vi "Measurement UI.vi"() -> ()   [LabVIEW 2021, in "adc_chToChIsolationMeasurement.lvlib"]
uses:
  adc_chToChIsolationMeasurement.lvlib
panel:
  in  "MeasGraphs":T1(tab)
  out "FreqDomainGraph":cluster{"f0":dbl, "df":dbl, "Spectrum":dbl[]}[](graph) caption="AC"
  out "TimeDomainGraph":waveform(dbl)[](graph) caption="AC"
  out "CrosstalkGraph":T2(graph)
  out "Time domain plot size":i32
  out "Spectrum plot size":i32
  out "dt":dbl
  out "t0":dbl
  out "df":dbl
  out "f0":dbl
  out "Time domain":dbl[](array[numeric])
  out "Spectrum":dbl[](array[numeric])
  in  "Interferer channel resource name":string
  out "Frequency":dbl
  out "Crosstalk":dbl
  out "Victim channel name":string
  out "Crosstalk waveform":dbl[](array[numeric])
  out "Frequency waveform":dbl[](array[numeric])
  in  "Victim channel resource name":string
  in  "Digital capture resource name":string
  out "MeasTable":string[][](table)
  in  "Interferer channel channel":i32 caption="CHANNEL"
  in  "MeasSettingsOptions":i32(listbox)
  in  "Digital capture":string="Digital capture"
  in  "Analog source interferer":string="Analog source interferer"
  in  "Analog source victim":string="Analog source victim"
  in  "ADC parameters":string="ADC parameters"
  in  "MeasSettings":bool
  in  "Interferer sweep type":u32(ring) caption="SWEEP TYPE" items=["Linear", "Logarithmic"]
  in  "Interferer number of steps":i32=10 caption="NUMBER OF STEPS"
  in  "Interferer stop frequency":dbl=160000.0 caption="STOP FREQUENCY" format="%#_6pHz"
  in  "Interferer amplitude":dbl=-1.0 caption="AMPLITUDE" format="%#_6pdB"
  in  "Interferer start frequency":dbl=2000.0 caption="START FREQUENCY" format="%#_6pHz"
  in  "InterfererResourceName":refnum<k15> caption="RESOURCE NAME"
  in  "Interferer channels":i32[](array[numeric])=[2] caption="INTERFERER CHANNELS"
  in  "Digital capture samples":u32=80000 caption="NUMBER OF SAMPLES"
  in  "Victim channel":i32 caption="VICTIM CHANNEL" min=0 max=100 step=1
  in  "Full scale range":dbl=10.0 caption="FULL SCALE RANGE" format="%#_6pV"
  in  "Digital capture sample rate":dbl=800000.0 caption="SAMPLE RATE" format="%#_6pS/s"
  in  "Victim amplitude":dbl=-1.0 caption="AMPLITUDE" format="%#_6pdB"
  in  "Victim frequency":dbl=1000.0 caption="FREQUENCY" format="%#_6pHz"
  in  "VictimResourceName":tag caption="RESOURCE NAME"
  in  "DPIResourceName":refnum<k15> caption="RESOURCE NAME"
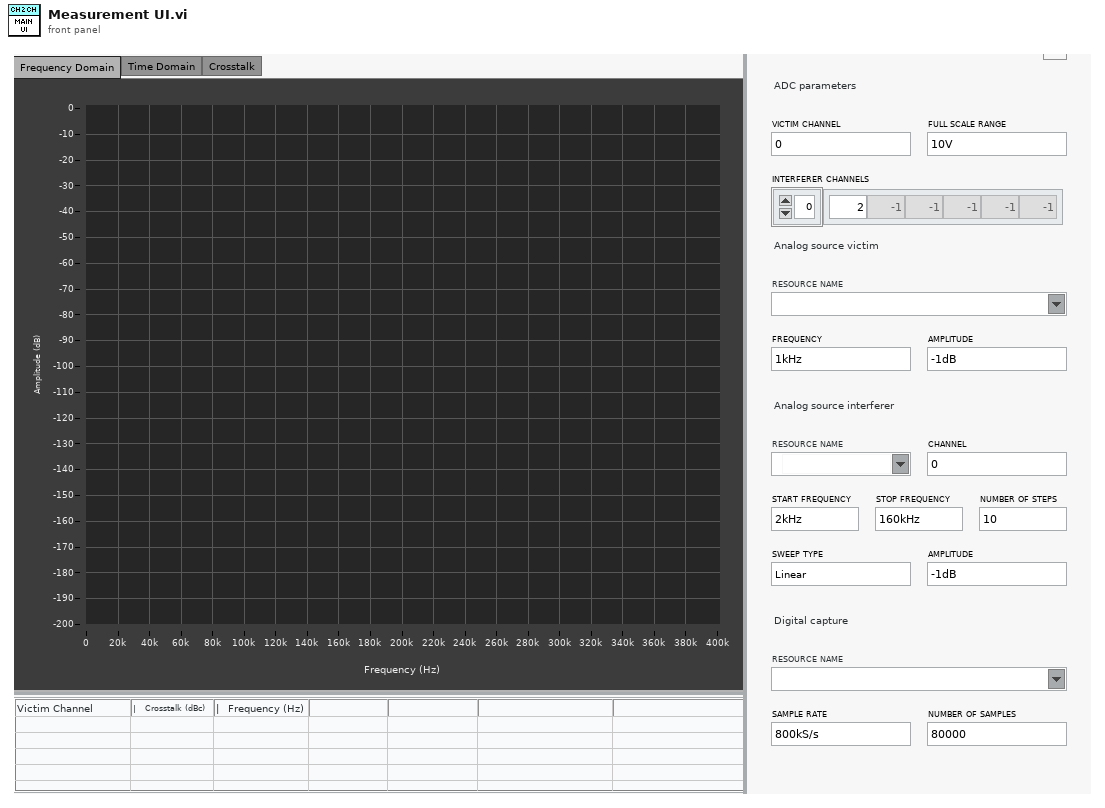
[diagram p1: front panel]
types:
  T1 = enum32{"Frequency Domain", "Time Domain", "Crosstalk", "Hidden Controls"}
  T2 = cluster{"Frequency waveform":dbl[], "Crosstalk waveform":dbl[]}
  T3 = enum16{"open", "replace", "create", "open or create", "replace or create", "replace or create with confirmation"}
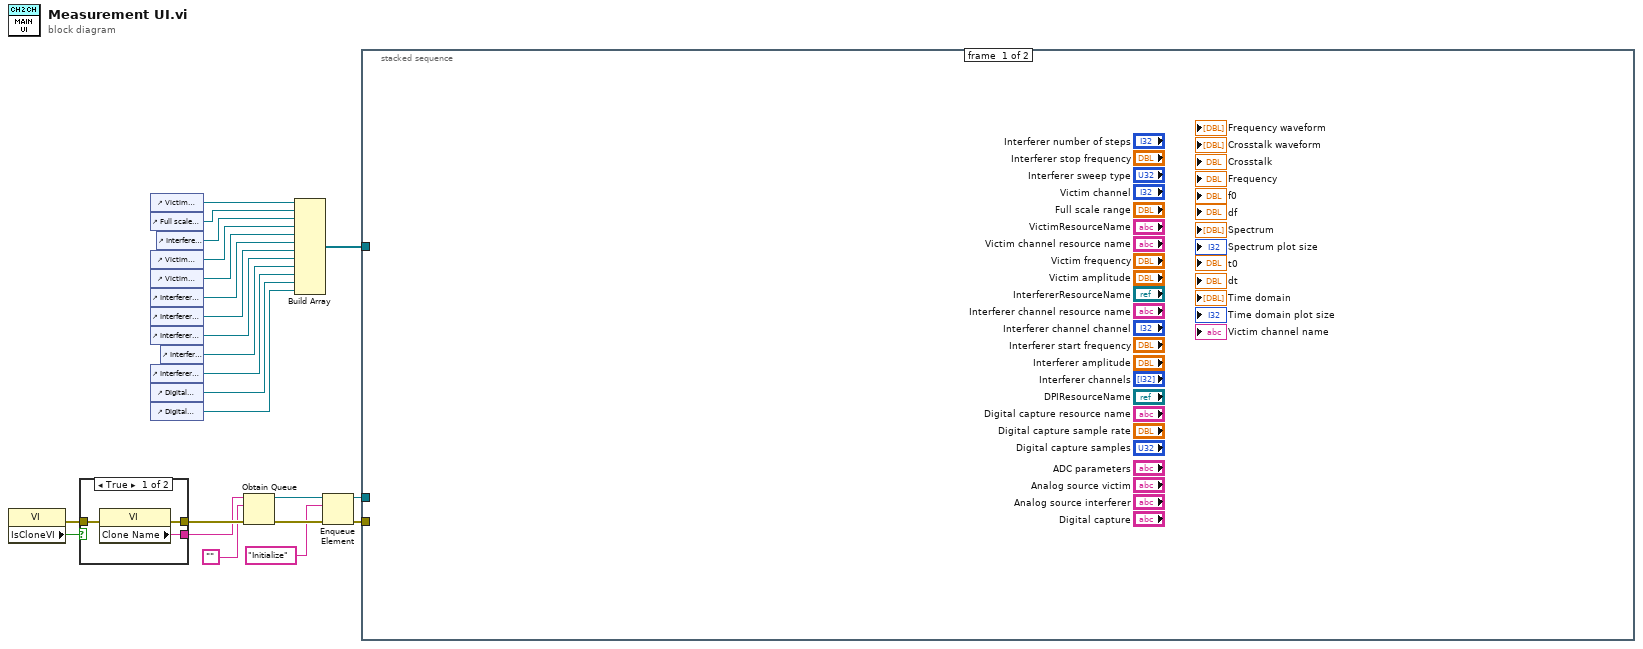
[diagram p0: block diagram]
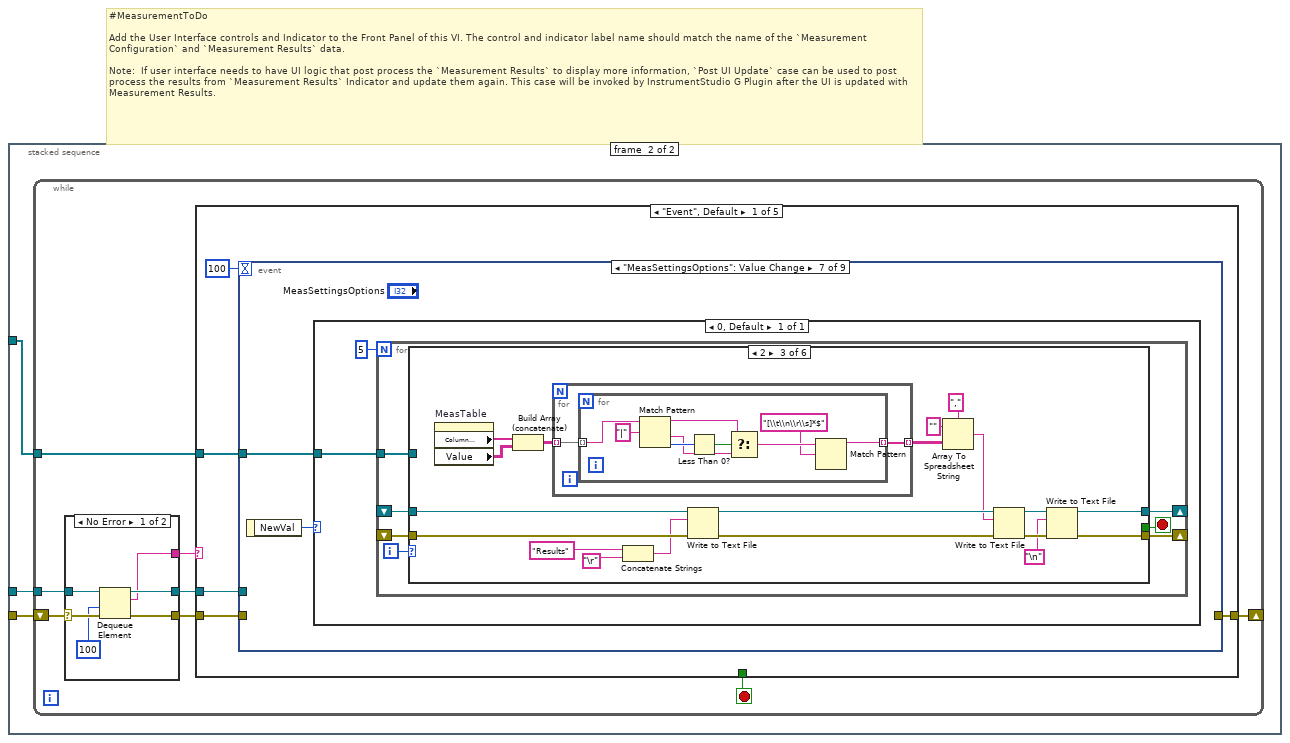
[diagram p2: hidden frame]
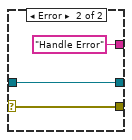
[diagram p3: hidden frame]
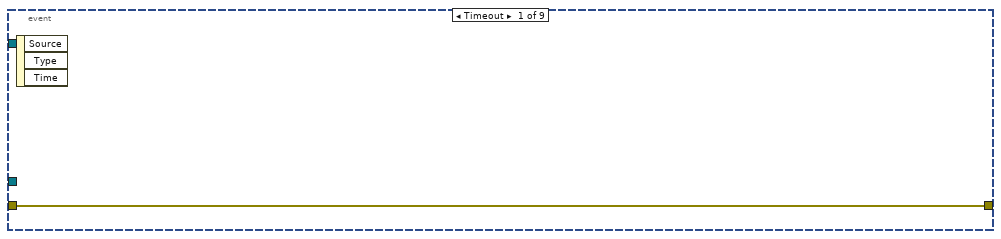
[diagram p4: hidden frame]
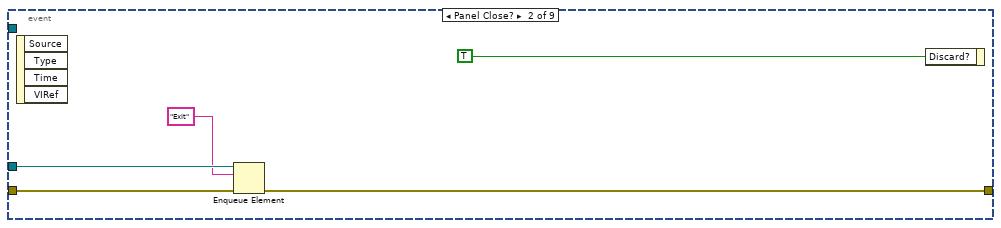
[diagram p5: hidden frame]
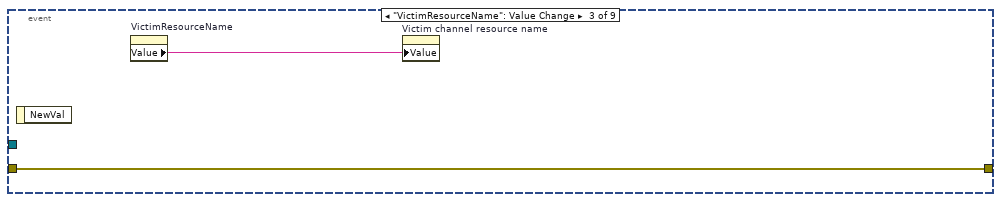
[diagram p6: hidden frame]
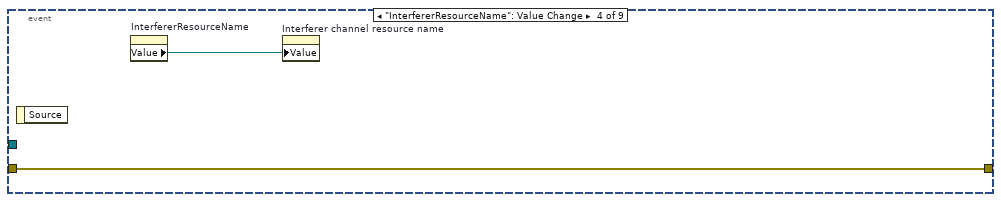
[diagram p7: hidden frame]
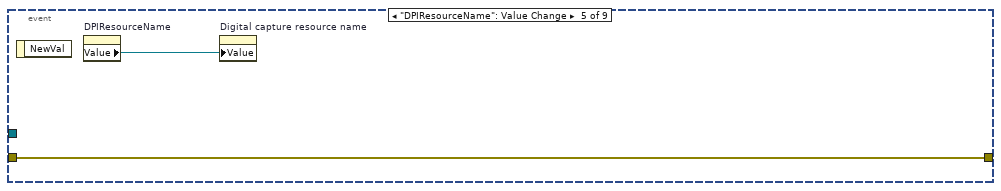
[diagram p8: hidden frame]
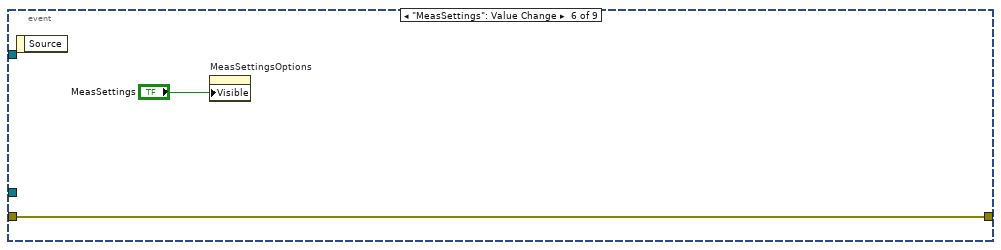
[diagram p9: hidden frame]
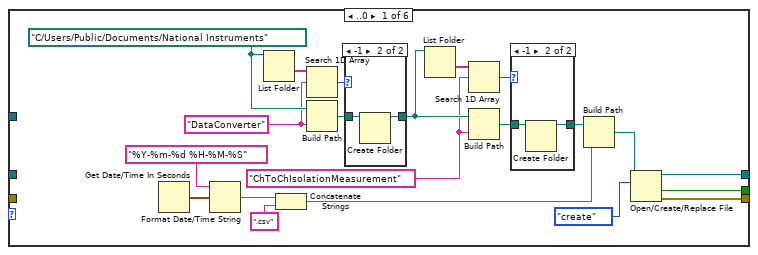
[diagram p10: hidden frame]
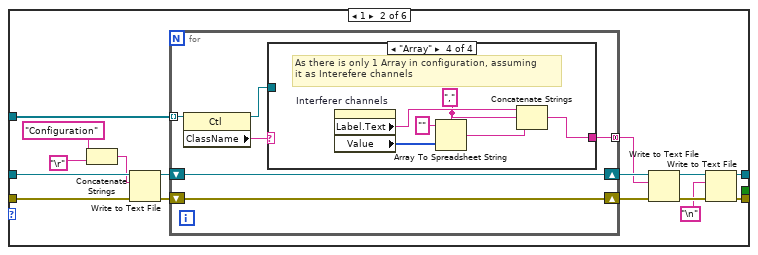
[diagram p13: hidden frame]
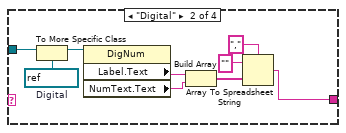
[diagram p15: hidden frame]
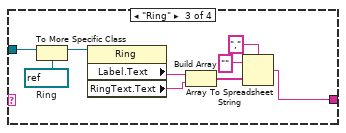
[diagram p16: hidden frame]
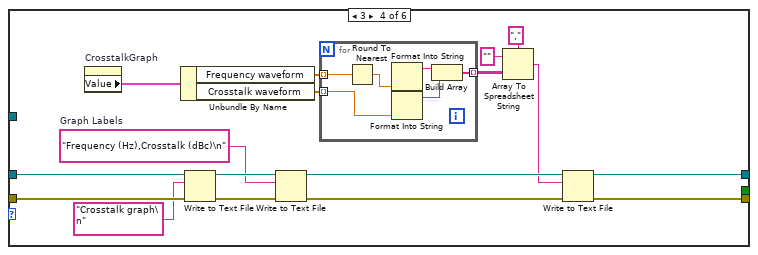
[diagram p17: hidden frame]
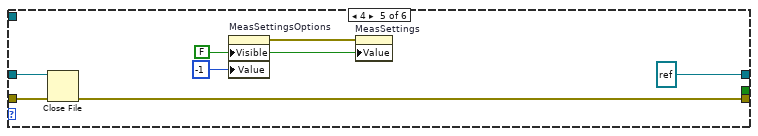
[diagram p18: hidden frame]
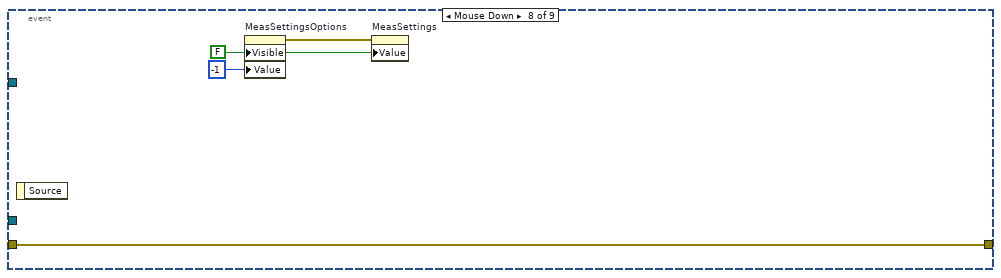
[diagram p20: hidden frame]
diagram:
  n1 = property class="VI"() -> (error out=w14:errorcluster, "IsCloneVI"=w15:bool)  [unwired: 2 in, 1 out]
  n2 = case shown="True" w15 {
    tunnel: [w26 w29] -> w23
    tunnel: [w25 w28] -> w22
    tunnel: w14 -> [w24 w27]
    frame True {
      n3 = property class="VI"(error in=w24) -> (error out=w26:errorcluster, "Clone Name"=w25:string)  [unwired: 1 in, 1 out]
    }
    frame False {
      n4 = property class="VI"(error in=w27) -> (error out=w29:errorcluster, "Name"=w28:string)  [unwired: 1 in, 1 out]
    }
  }
  n5 = control-ref of="Victim channel"() -> (w2:refnum<vi>)
  n6 = control-ref of="Full scale range"() -> (w3:refnum<vi>)
  n7 = control-ref of="Victim frequency"() -> (w5:refnum<vi>)
  n8 = control-ref of="Victim amplitude"() -> (w6:refnum<vi>)
  n9 = control-ref of="Interferer start frequency"() -> (w7:refnum<vi>)
  n10 = control-ref of="Interferer stop frequency"() -> (w8:refnum<vi>)
  n11 = control-ref of="Interferer number of steps"() -> (w9:refnum<vi>)
  n12 = control-ref of="Interferer amplitude"() -> (w11:refnum<vi>)
  n13 = control-ref of="Digital capture sample rate"() -> (w12:refnum<vi>)
  n14 = control-ref of="Digital capture samples"() -> (w13:refnum<vi>)
  n15 = control-ref of="Interferer channels"() -> (w4:refnum<vi>)
  n16 = control-ref of="Interferer sweep type"() -> (w10:refnum<vi>)
  n17 = Obtain Queue(name (unnamed)=w22, element data type="", error in (no error)=w23) -> (queue out=w19:refnum<queue>, error out=w21:errorcluster)  [unwired: 2 in, 1 out]
  n18 = Build Array(w2, w3, w4, w5, w6, w7, w8, w9, w10, w11, w12, w13) -> (w1:refnum<vi>[])
  n19 = Enqueue Element(queue=w19, element="Initialize", error in (no error)=w21) -> (queue out=w18:refnum<queue>, error out=w20:errorcluster)  [unwired: 1 in, 1 out]
  n20 = stacked-sequence {
    tunnel: w20 -> [_ w32]
    tunnel: w18 -> [_ w31]
    tunnel: w1 -> [_ w30]
    frame #0 {
    }
    frame #1 {
      # "#MeasurementToDo  \n\nAdd the User Interface controls and Indicator to the Front Panel of this VI. The control and indicator label name should match the name of the `Measurement Configuration` and `Measurement Results` data.\n\nNote:  If user interface needs to have UI logic that post process the `Measurement Results` to display more information, `Post UI Update` case can be used to post process the results from `Measurement Results` Indicator and update them again. This case will be invoked by InstrumentStudio G Plugin after the UI is updated with Measurement Results."
      n21 = while {
        shift-right: [w35] -> _
        shift-left: w32 -> [w40]
        tunnel: w31 -> [w38]
        tunnel: w30 -> [w33]
        stop <- w34 stop-if-true
        n22 = case shown="No Error" w40 {
          selector: w40 -> [w46 w49]
          tunnel: [w45 w49] -> w39
          tunnel: w38 -> [w44 w48]
          tunnel: [w43 w48] -> w37
          tunnel: [w42 "Handle Error"] -> w36
          frame No Error {
            n23 = Dequeue Element(queue=w44, timeout in ms (-1)=100, error in (no error)=w46) -> (queue out=w43:refnum<queue>, element=w42:string, error out=w45:errorcluster)  [unwired: 1 out]
          }
          frame Error {
          }
        }
        n24 = case shown="\"Event\", Default" w36 {
          tunnel: w39 -> [w53 w240 w268 w292 w293]
          tunnel: w37 -> [w51 _ _ w290 _]
          tunnel: [w54 w240 w268 w287 w293] -> w35
          tunnel: [_ _ _ TRUE _] -> w34
          tunnel: w33 -> [w50 _ _ _ _]
          frame "Event", Default {
            n25 = event shown="[6] \"MeasSettingsOptions\": Value Change" {
              selector: _ -> [_ _ _ _ _ _ _ _ _]
              dyn-events: _ -> [_ _ _ _ _ _ _ _ _]
              timeout: 100 -> [_ _ _ _ _ _ _ _ _]
              tunnel: [w55 w58 w62 w64 w65 w67 _ w218 w219] -> w54
              tunnel: w53 -> [w55 w59 w62 w64 w65 w67 _ w218 w219]
              tunnel: w51 -> [_ w57 _ _ _ _ _ _ _]
              tunnel: w50 -> [_ _ _ _ _ _ w69 _ _]
              event Timeout {
                n26 = event-data() -> ()  [unwired: 1 in, 3 out]
              }
              event Panel Close? {
                n27 = event-data() -> ()  [unwired: 1 in, 4 out]
                n28 = Enqueue Element(queue=w57, element="Exit", error in (no error)=w59) -> (error out=w58:errorcluster)  [unwired: 1 in, 2 out]
                n29 = event-data("Discard?"=TRUE) -> ()  [unwired: 1 in, 1 out]
              }
              event "VictimResourceName": Value Change {
                n30 = event-data() -> ()  [unwired: 1 in, 1 out]
                n31 = property on="VictimResourceName" class="DAQmxName"() -> ("Value"=w61:string)  [unwired: 2 in, 2 out]
                n32 = property on="Victim channel resource name" class="Str"("Value"=w61) -> ()  [unwired: 2 in, 2 out]
              }
              event "InterfererResourceName": Value Change {
                n33 = event-data() -> ()  [unwired: 1 in, 1 out]
                n34 = property on="InterfererResourceName" class="IVIName"() -> ("Value"=w63:refnum<k15>)  [unwired: 2 in, 2 out]
                n35 = property on="Interferer channel resource name" class="Str"("Value"=w63) -> ()  [unwired: 2 in, 2 out]
              }
              event "DPIResourceName": Value Change {
                n36 = event-data() -> ()  [unwired: 1 in, 1 out]
                n37 = property on="DPIResourceName" class="IVIName"() -> ("Value"=w66:refnum<k15>)  [unwired: 2 in, 2 out]
                n38 = property on="Digital capture resource name" class="Str"("Value"=w66) -> ()  [unwired: 2 in, 2 out]
              }
              event "MeasSettings": Value Change {
                n39 = event-data() -> ()  [unwired: 1 in, 1 out]
                n40 = property on="MeasSettingsOptions" class="LstBox (strict)"("Visible"="MeasSettings") -> ()  [unwired: 2 in, 2 out]
              }
              event "MeasSettingsOptions": Value Change {
                n41 = event-data() -> ("NewVal"=w70:i32)  [unwired: 1 in]
                n42 = case shown="0, Default" w70 {
                  tunnel: w69 -> [w72]
                  frame 0, Default {
                    n43 = for {
                      N: 5 -> [_]
                      shift-right: [w77] -> _
                      shift-left: _ -> [w76]
                      shift-right: [w75] -> _
                      shift-left: _ -> [w74]
                      tunnel: w72 -> [w73]
                      i -> [w79]
                      stop <- w78 stop-if-true
                      n44 = case shown="2" w79 {
                        tunnel: [w93 _ _ _ _ _] -> w78
                        tunnel: [w99 w110 w158 w185 refnum<file> refnum ("refnum out") w214] -> w77
                        tunnel: w76 -> [_ w121 w171 w199 w209 w214]
                        tunnel: [w92 w109 w157 w184 w207 w213] -> w75
                        tunnel: w74 -> [_ w119 w170 w198 w208 w213]
                        tunnel: w73 -> [_ w107 _ _ _ _]
                        frame ..0 {
                          w88 = "ChToChIsolationMeasurement" ("prompt")
                          w95 = "DataConverter" ("prompt")
                          w98 = path "C:/Users/Public/Documents/National Instruments" ("base path")
                          n45 = Get Date/Time In Seconds() -> (seconds since 1Jan1904=w85:timestamp)
                          n46 = Format Date/Time String(time format string (%c)="%Y-%m-%d %H-%M-%S", seconds (now)=w85) -> (date/time string=w84:string)  [unwired: 1 in]
                          n47 = List Folder(path=w98) -> (folder names=w96:string[])  [unwired: 3 in, 3 out]
                          n48 = Concatenate Strings(w84, ".csv" ("string")) -> (w81:string)
                          n49 = Search 1D Array(1D array=w96, element=w95) -> (index of element=w94:i32)  [unwired: 1 in]
                          n50 = Build Path(base path=w98, name or relative path=w95) -> (appended path=w97:path)
                          n51 = case shown="-1" w94 {
                            tunnel: w97 -> [w104 w106]
                            tunnel: [w104 w105] -> w89
                            frame Default {
                            }
                            frame -1 {
                              n52 = Create Folder(path (use dialog)=w106) -> (created path=w105:path)  [unwired: 2 in, 2 out]
                            }
                          }
                          n53 = List Folder(path=w89) -> (folder names=w91:string[])  [unwired: 3 in, 3 out]
                          n54 = Search 1D Array(1D array=w91, element=w88) -> (index of element=w90:i32)  [unwired: 1 in]
                          n55 = Build Path(base path=w89, name or relative path=w88) -> (appended path=w87:path)
                          n56 = case shown="-1" w90 {
                            tunnel: w87 -> [w101 w103]
                            tunnel: [w101 w102] -> w82
                            frame Default {
                            }
                            frame -1 {
                              n57 = Create Folder(path (use dialog)=w103) -> (created path=w102:path)  [unwired: 2 in, 2 out]
                            }
                          }
                          n58 = Build Path(base path=w82, name or relative path=w81) -> (appended path=w80:path)
                          n59 = Open/Create/Replace File(file path (use dialog)=w80, operation (0:open)=T3."create") -> (refnum out=w99:refnum<file>, cancelled=w93:bool, error out=w92:errorcluster)  [unwired: 4 in]
                        }
                        frame 1 {
                          n60 = Concatenate Strings("Configuration" ("format string"), "\r") -> (w116:string)
                          n61 = Write to Text File(file (use dialog)=w121, text=w116, error in=w119) -> (refnum out=w122:refnum<file>, error out=w120:errorcluster)  [unwired: 1 in, 1 out]
                          n62 = for {
                            tunnel: w107 -> [w124] mode=indexing
                            shift-right: [w128] -> w115
                            shift-left: w122 -> [w128]
                            shift-right: [w127] -> w113
                            shift-left: w120 -> [w127]
                            tunnel: [w126] -> w111 mode=concatenating
                            n63 = property class="Ctl"(reference=w124) -> (reference out=w125:refnum<vi>, "ClassName"=w123:string)  [unwired: 1 in, 1 out]
                            n64 = case shown="\"Array\"" w123 {
                              tunnel: [_ w132 w141 w149] -> w126
                              tunnel: w125 -> [_ w130 w139 _]
                              frame Default {
                              }
                              frame "Digital" {
                                w129 = refnum<vi> refnum  # Digital
                                n65 = To More Specific Class(target class=w129, reference=w130) -> (specific class reference=w131:refnum<vi>)  [unwired: 1 in, 1 out]
                                n66 = property class="DigNum"(reference=w131) -> ("Label.Text"=w137:string, "NumText.Text"=w136:string)  [unwired: 1 in, 2 out]
                                n67 = Build Array(w137, w136) -> (w133:string[])
                                n68 = Array To Spreadsheet String(delimiter (Tab)=",", array=w133, 3:"" ("format string")) -> (spreadsheet string=w132:string)
                              }
                              frame "Ring" {
                                w138 = refnum<vi> refnum  # Ring
                                n69 = To More Specific Class(target class=w138, reference=w139) -> (specific class reference=w140:refnum<vi>)  [unwired: 1 in, 1 out]
                                n70 = property class="Ring"(reference=w140) -> ("Label.Text"=w146:string, "RingText.Text"=w145:string)  [unwired: 1 in, 2 out]
                                n71 = Build Array(w146, w145) -> (w142:string[])
                                n72 = Array To Spreadsheet String(delimiter (Tab)=",", array=w142, 3:"" ("format string")) -> (spreadsheet string=w141:string)
                              }
                              frame "Array" {
                                w148 = "," ("delimiter (Tab)")
                                # "As there is only 1 Array in configuration, assuming\nit as Interefere channels"
                                n73 = property on="Interferer channels" class="Arr (strict)"() -> ("Label.Text"=w152:string, "Value"=w151:i32[])  [unwired: 2 in, 2 out]
                                n74 = Array To Spreadsheet String(delimiter (Tab)=w148, array=w151, 3:"" ("format string")) -> (spreadsheet string=w147:string)
                                n75 = Concatenate Strings(w152, w148, w147) -> (w149:string)
                              }
                            }
                          }
                          n76 = Write to Text File(file (use dialog)=w115, text=w111, error in=w113) -> (refnum out=w114:refnum<file>, error out=w112:errorcluster)  [unwired: 1 in, 1 out]
                          n77 = Write to Text File(file (use dialog)=w114, text="\n", error in=w112) -> (refnum out=w110:refnum<file>, error out=w109:errorcluster)  [unwired: 1 in, 1 out]
                        }
                        frame 2 {
                          n78 = property on="MeasTable" class="Tbl (strict)"() -> ("Column Headers[]"=w168:string[], "Value"=w167:string[][])  [unwired: 2 in, 2 out]
                          n79 = Build Array (concatenate)(w168, w167) -> (w166:string[][])
                          n80 = for {
                            tunnel: w166 -> [w173] mode=indexing
                            tunnel: [w172] -> w165 mode=indexing
                            n81 = for {
                              tunnel: w173 -> [w175] mode=indexing
                              tunnel: [w174] -> w172 mode=indexing
                              n82 = Match Pattern(string=w175, regular expression="|") -> (before substring=w179:string, after substring=w178:string, offset past match=w181:i32)  [unwired: 1 in, 1 out]
                              n83 = Less Than 0?(x=w181) -> (x < 0?=w180:bool)
                              n84 = Select(t=w179, s=w180, f=w178) -> (s? t:f=w177:string)
                              n85 = Match Pattern(string=w177, regular expression="[\\t\\n\\r\\s]*$") -> (before substring=w174:string)  [unwired: 1 in, 3 out]
                            }
                          }
                          n86 = Concatenate Strings("Results" ("element"), "\r") -> (w153:string)
                          n87 = Write to Text File(file (use dialog)=w171, text=w153, error in=w170) -> (refnum out=w169:refnum<file>, error out=w161:errorcluster)  [unwired: 1 in, 1 out]
                          n88 = Array To Spreadsheet String(delimiter (Tab)=",", array=w165, 3:"" ("format string")) -> (spreadsheet string=w162:string)
                          n89 = Write to Text File(file (use dialog)=w169, text=w162, error in=w161) -> (refnum out=w160:refnum<file>, error out=w159:errorcluster)  [unwired: 1 in, 1 out]
                          n90 = Write to Text File(file (use dialog)=w160, text="\n", error in=w159) -> (refnum out=w158:refnum<file>, error out=w157:errorcluster)  [unwired: 1 in, 1 out]
                        }
                        frame 3 {
                          w183 = "Frequency (Hz),Crosstalk (dBc)\n"  # Graph Labels
                          n91 = property on="CrosstalkGraph" class="XYGraph (strict)"() -> ("Value"=w188:T2)  [unwired: 2 in, 2 out]
                          n92 = Unbundle By Name(w188) -> ("Frequency waveform"=w189:dbl[], "Crosstalk waveform"=w190:dbl[])
                          n93 = Write to Text File(file (use dialog)=w199, text="Crosstalk graph\n" ("string"), error in=w198) -> (refnum out=w197:refnum<file>, error out=w196:errorcluster)  [unwired: 1 in, 1 out]
                          n94 = Write to Text File(file (use dialog)=w197, text=w183, error in=w196) -> (refnum out=w195:refnum<file>, error out=w194:errorcluster)  [unwired: 1 in, 1 out]
                          n95 = for {
                            tunnel: w189 -> [w201] mode=indexing
                            tunnel: w190 -> [w202] mode=indexing
                            tunnel: [w203] -> w191 mode=indexing
                            n96 = Round To Nearest(number=w201) -> (nearest integer value=w200:dbl)
                            n97 = Format Into String(w200) -> (resulting string=w204:string)  [unwired: 3 in, 1 out]
                            n98 = Format Into String(w202) -> (resulting string=w205:string)  [unwired: 3 in, 1 out]
                            n99 = Build Array(w204, w205) -> (w203:string[])
                          }
                          n100 = Array To Spreadsheet String(delimiter (Tab)=",", array=w191, 3:"" ("format string")) -> (spreadsheet string=w187:string)
                          n101 = Write to Text File(file (use dialog)=w195, text=w187, error in=w194) -> (refnum out=w185:refnum<file>, error out=w184:errorcluster)  [unwired: 1 in, 1 out]
                        }
                        frame 4 {
                          w211 = FALSE ("Visible")
                          n102 = Close File(refnum=w209, error in=w208) -> (error out=w207:errorcluster)  [unwired: 1 out]
                          n103 = property on="MeasSettingsOptions" class="LstBox (strict)"("Visible"=w211, "Value"=-1 ("MeasSettingsOptions")) -> (error out=w212:errorcluster)  [unwired: 2 in, 1 out]
                          n104 = property on="MeasSettings" class="Bool (strict)"(error in=w212, "Value"=w211) -> ()  [unwired: 1 in, 2 out]
                        }
                        frame Default {
                        }
                      }
                    }
                  }
                }
              }
              event Mouse Down {
                w216 = FALSE ("Visible")
                n105 = event-data() -> ()  [unwired: 1 in, 1 out]
                n106 = property on="MeasSettingsOptions" class="LstBox (strict)"("Visible"=w216, "Value"=-1 ("MeasSettingsOptions")) -> (error out=w217:errorcluster)  [unwired: 2 in, 1 out]
                n107 = property on="MeasSettings" class="Bool (strict)"(error in=w217, "Value"=w216) -> ()  [unwired: 1 in, 2 out]
              }
              event "FreqDomainGraph", "Time domain", "CrosstalkGraph": Shortcut Menu Selection (User) {
                n108 = event-data() -> ("ItemTag"=w223:string)  [unwired: 1 in]
                n109 = case shown="\"ZOOM_TO_RECTANGLE\", Default" w223 {
                  tunnel: [2 ("Palette:Active Tool") 3 ("Palette:Active Tool") 4 ("Palette:Active Tool") 5 ("Palette:Active Tool") 1 ("Palette:Active Tool")] -> w220
                  frame "ZOOM_TO_RECTANGLE", Default {
                  }
                  frame "X_ZOOM" {
                  }
                  frame "Y_ZOOM" {
                  }
                  frame "ZOOM_TO_FIT" {
                  }
                  frame "PANNING_TOOL" {
                  }
                }
                n110 = case shown="\"Frequency Domain\", Default" "MeasGraphs" {
                  tunnel: [w224 w225 w226] -> w221
                  frame "Frequency Domain", Default {
                    n111 = control-ref of="FreqDomainGraph"() -> (w224:refnum<vi>)
                  }
                  frame "Time Domain" {
                    n112 = control-ref of="TimeDomainGraph"() -> (w225:refnum<vi>)
                  }
                  frame "Crosstalk" {
                    n113 = control-ref of="CrosstalkGraph"() -> (w226:refnum<vi>)
                  }
                }
                n114 = property class="WFGraph"(reference=w221, "ActPaletteTool"=w220) -> ()  [unwired: 1 in, 2 out]
              }
            }
          }
          frame "Initialize" {
            w232 = 2 ("Palette:Active Tool")
            w237 = string[] ["Export data"] ("Item Names")
            w239 = "<Select Device>"
            n115 = property on="VictimResourceName" class="DAQmxName"("Value"=w239) -> ()  [unwired: 2 in, 2 out]
            n116 = property on="DPIResourceName" class="IVIName"("Value"=w239) -> ()  [unwired: 2 in, 2 out]
            n117 = property on="InterfererResourceName" class="IVIName"("Value"=w239) -> ()  [unwired: 2 in, 2 out]
            n118 = property on="MeasGraphs" class="TabCtl (strict)"("Value"=T1."Crosstalk" ("MeasGraphs")) -> ()  [unwired: 2 in, 2 out]
            n119 = property on="MeasSettingsOptions" class="LstBox (strict)"("Item Names"=w237, "Value"=-1 ("MeasSettingsOptions"), "Visible"=FALSE, "Disabled Items"=i32[] []) -> ()  [unwired: 2 in, 2 out]
            n120 = property on="FreqDomainGraph" class="WFGraph (strict)"("ActPaletteTool"=w232) -> ()  [unwired: 2 in, 2 out]
            n121 = for {
              tunnel: w237 -> [_] mode=indexing
              i -> [w242]
              n122 = property on="MeasSettingsOptions" class="LstBox (strict)"("Active Row"=w242, "Cell Height"=30 ("Active Row:Cell Height")) -> ()  [unwired: 2 in, 2 out]
            }
            n123 = property on="TimeDomainGraph" class="WFGraph (strict)"("ActPaletteTool"=w232) -> ()  [unwired: 2 in, 2 out]
            n124 = property on="MeasTable" class="Tbl (strict)"("Column Headers[]"=string[] ["Victim Channel", "|   Crosstalk (dBc)", "|   Frequency (Hz)"] ("Column Header Strings[]")) -> ()  [unwired: 2 in, 2 out]
            n125 = property on="CrosstalkGraph" class="XYGraph (strict)"("ActPaletteTool"=w232) -> ()  [unwired: 2 in, 2 out]
          }
          frame "Post UI Update" {
            # "This case will be triggered, after framework updates the User interface with result values."
            n126 = local read "Frequency"() -> (w266:dbl)
            n127 = local read "Frequency waveform"() -> (w258:dbl[])
            n128 = local read "Crosstalk"() -> (w267:dbl)
            n129 = local read "Crosstalk waveform"() -> (w257:dbl[])
            n130 = local read "Victim channel name"() -> (w259:string)
            n131 = Build Array(w267, w266) -> (w265:dbl[])
            n132 = for {
              tunnel: w265 -> [w282] mode=indexing
              tunnel: "|   " ("initial string") -> [w283]
              tunnel: "%#_6p" ("initial string") -> [w284]
              tunnel: [w285] -> w262 mode=indexing
              n133 = Format Into String(format string=w284, initial string=w283, w282) -> (resulting string=w285:string)  [unwired: 1 in, 1 out]
            }
            n134 = Bundle("Frequency waveform"=w258, "Crosstalk waveform"=w257) -> (→"CrosstalkGraph":T2)  [unwired: 1 in]
            n135 = local read "Time domain plot size"() -> (w245:i32)
            n136 = local read "Spectrum plot size"() -> (w252:i32)
            n137 = local read "Time domain"() -> (w247:dbl[])
            n138 = local read "Spectrum"() -> (w253:dbl[])
            n139 = Build Array (concatenate)(w259, w262) -> (w261:string[])
            n140 = Build Array(w261) -> (→"MeasTable":string[][])
            n141 = Array Size(array=w253) -> (size(s)=w255:i32)
            n142 = Array Size(array=w247) -> (size(s)=w246:i32)
            n143 = local read "df"() -> (w250:dbl)
            n144 = local read "dt"() -> (w243:dbl)
            n145 = local read "f0"() -> (w251:dbl)
            n146 = Quotient & Remainder(x=w255, y=w252) -> (floor(x/y)=w254:i32)  [unwired: 1 out]
            n147 = Quotient & Remainder(x=w246, y=w245) -> (floor(x/y)=w248:i32)  [unwired: 1 out]
            n148 = for {
              N: w254 -> [_]
              shift-right: [w280] -> _
              shift-left: w253 -> [w281]
              tunnel: w252 -> [w279]
              tunnel: w251 -> [w278]
              tunnel: w250 -> [w277]
              tunnel: [w275] -> w249 mode=indexing
              n149 = Delete From Array(array=w281, length=w279) -> (deleted portion=w276:dbl[], array with subset deleted=w280:dbl[])  [unwired: 1 in]
              n150 = Bundle("f0"=w278, "df"=w277, "Spectrum"=w276) -> (w275:cluster{"f0":dbl, "df":dbl, "Spectrum":dbl[]})  [unwired: 1 in]
            }
            "FreqDomainGraph" <- w249
            n151 = for {
              N: w248 -> [_]
              shift-right: [w273] -> _
              shift-left: w247 -> [w274]
              tunnel: w245 -> [w272]
              tunnel: [w270] -> w244 mode=indexing
              tunnel: w243 -> [w269]
              n152 = Delete From Array(array=w274, length=w272) -> (deleted portion=w271:dbl[], array with subset deleted=w273:dbl[])  [unwired: 1 in]
              n153 = Bundle By Name("dt"=w269, "Y"=w271) -> (w270:waveform(dbl))  [unwired: 1 in]
            }
            "TimeDomainGraph" <- w244
          }
          frame "Exit" {
            # "This case is triggered to close the User Interface from framework"
            n154 = Flush Queue(queue=w290, error in (no error)=w292) -> (queue out=w289:refnum<queue>, error out=w288:errorcluster)  [unwired: 1 out]
            n155 = Release Queue(queue=w289, force destroy? (F)=TRUE, error in (no error)=w288) -> (error out=w287:errorcluster)  [unwired: 2 out]
          }
          frame "Handle Error" {
          }
        }
      }
    }
  }
